vi "Dynamixel Motor Setup.vi"() -> ()   [LabVIEW 2016]
doc: "This example is designed for configuring attributes typically set on a dynamixel motor before first use."
uses:
  <instrlib>/Dynamixel Motor/Public/Motor Operation/Low Level/Alarm Setting.ctl
  <instrlib>/Dynamixel Motor/Public/Motor Operation/Low Level/Baud Setting.ctl
  <instrlib>/Dynamixel Motor/Dynamixel Motor.lvlib
panel:
  out "Searching for motor":bool
  in  "Tab Control":enum32{"Port setup", "Auto-detect settings"}(tab)
  in  "VISA resource name":refnum<visa-resource-name>
  in  "Baud rate (57600 bps)":T1=34 items=["1,000,000 bps"=1, "500,000 bps"=3, "400,000 bps"=4, "250,000 bps"=7, "200,000 bps"=9, "115200 bps"=16, "57600 bps"=34, "19200 bps"=103, "9600 bps"=207]
  in  "Force Baud Rate (True)":bool=TRUE
  in  "Search Timeout (10000 ms)":u32=10000
  in  "Starting ID (0)":u8
  in  "Ending ID (253)":u8=253
  in  "stop":bool
  out "Current angles":cluster{dbl, dbl, dbl}(knob)={0.0, 0.0, 300.0} scale=0.0..300.0
  in  "Counter-Clockwise Limit":dbl=300.0
  in  "Clockwise Limit":dbl
  out "Current Safety Limits":T2={"Temperature Limit (C)"=80, "Low Voltage Limit (V)"=6.0, "High Voltage Limit (V)"=19.0, "Maximum Torque%"=100.0} {"Maximum Torque%" min=0.0 max=100.0; "High Voltage Limit (V)" min=5.0 max=25.0; "Low Voltage Limit (V)" min=5.0 max=25.0; "Temperature Limit (C)" max=150 step=1}
  in  "Desired Safety Limits":T2={"Temperature Limit (C)"=80, "Low Voltage Limit (V)"=6.0, "High Voltage Limit (V)"=19.0, "Maximum Torque%"=100.0} {"Maximum Torque%" min=0.0 max=100.0; "High Voltage Limit (V)" min=5.0 max=25.0; "Low Voltage Limit (V)" min=5.0 max=25.0; "Temperature Limit (C)" max=150 step=1}
  in  "Apply new settings":bool
  out "Current Alarm Settings":cluster{"LED Alarm":T3, "Shutdown Alarm":T3}={"LED Alarm"={"Input Voltage"=FALSE, "Angle Limit"=FALSE, "Overheating "=TRUE, "Range"=FALSE, "Checksum"=FALSE, "Overload"=TRUE, "Instruction"=FALSE}, "Shutdown Alarm"={"Input Voltage"=FALSE, "Angle Limit"=FALSE, "Overheating "=TRUE, "Range"=FALSE, "Checksum"=FALSE, "Overload"=TRUE, "Instruction"=FALSE}}
  in  "Desired Alarm Settings":cluster{"LED Alarm":T3, "Shutdown Alarm":T3}={"LED Alarm"={"Input Voltage"=FALSE, "Angle Limit"=FALSE, "Overheating "=TRUE, "Range"=FALSE, "Checksum"=FALSE, "Overload"=TRUE, "Instruction"=FALSE}, "Shutdown Alarm"={"Input Voltage"=FALSE, "Angle Limit"=FALSE, "Overheating "=TRUE, "Range"=FALSE, "Checksum"=FALSE, "Overload"=TRUE, "Instruction"=FALSE}}
  in  "Change ID":bool
  out "Current ID":u8
  in  "New ID":u8
  # "(c) 2011-2012  National Instruments.  ALL RIGHTS RESERVED."
  # "This example is designed for \nconfiguring attributes typically set \non a Dynamixel motor before first \nuse.  \n\n1. Connect only one motor to the\nserial communications line. \n2. Choose the serial communication \nsettings and optionally the auto \ndetect settings.  \n3. Run the VI.\n4. Change the ID if desired.\n5. Enter other desired settings and\nclick Apply new settings.\n6. Stop the VI and repeat for each\nmotor you wish to configure."
  # "Clockwise Limit"
  # "Motor Position"
  # "Counter-Clockwise Limit"
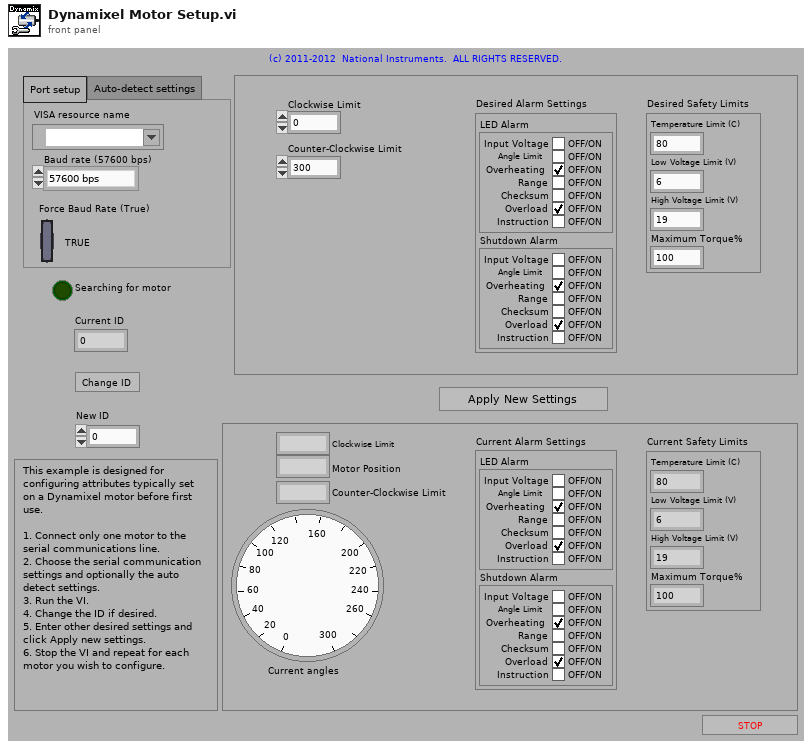
[diagram p1: front panel]
types:
  T1 = typedef "Dynamixel Motor.lvlib/Baud Setting.ctl" = u8
  T2 = cluster{"Temperature Limit (C)":u8, "Low Voltage Limit (V)":dbl, "High Voltage Limit (V)":dbl, "Maximum Torque%":dbl}
  T3 = typedef "Dynamixel Motor.lvlib/Alarm Setting.ctl" = cluster{"Input Voltage":bool, "Angle Limit":bool, "Overheating ":bool, "Range":bool, "Checksum":bool, "Overload":bool, "Instruction":bool}
  T4 = cluster{"Boolean array[0]":bool, "Boolean array[1]":bool, "Boolean array[2]":bool, "Boolean array[3]":bool, "Boolean array[4]":bool, "Boolean array[5]":bool, "Boolean array[6]":bool}
  T5 = cluster{"Boolean array":cluster{"Boolean array[0]":bool, "Boolean array[1]":bool, "Boolean array[2]":bool, "Boolean array[3]":bool, "Boolean array[4]":bool, "Boolean array[5]":bool, "Boolean array[6]":bool}, "Boolean array":cluster{"Boolean array[0]":bool, "Boolean array[1]":bool, "Boolean array[2]":bool, "Boolean array[3]":bool, "Boolean array[4]":bool, "Boolean array[5]":bool, "Boolean array[6]":bool}}
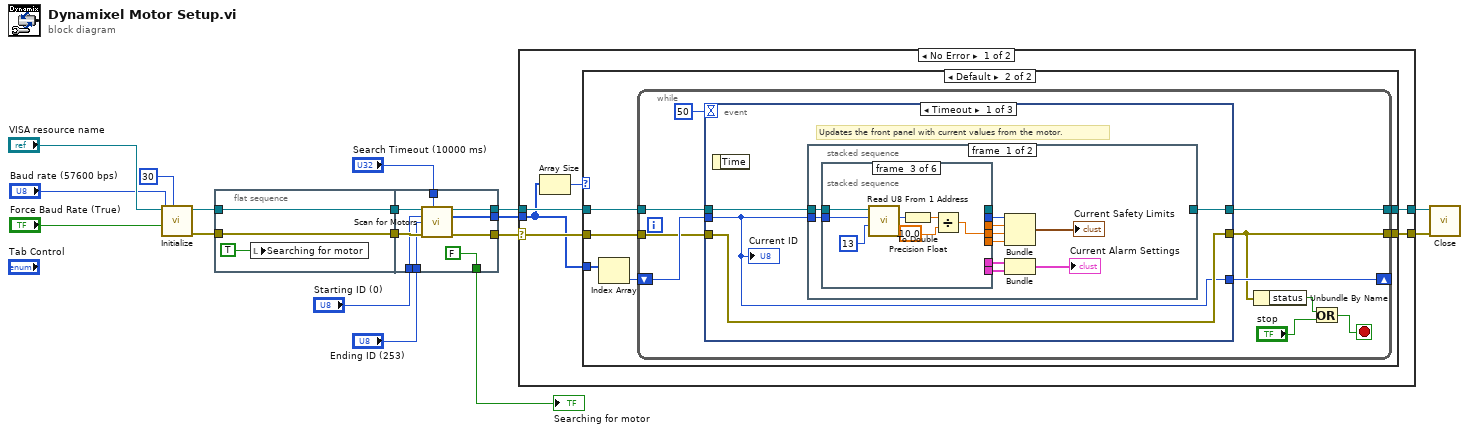
[diagram p0: block diagram]
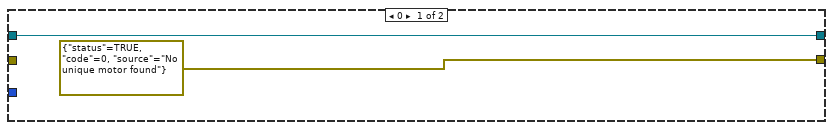
[diagram p2: hidden frame]
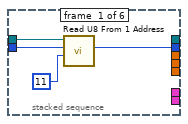
[diagram p3: hidden frame]
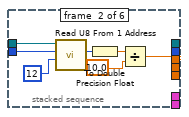
[diagram p4: hidden frame]
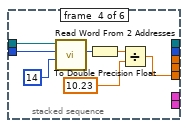
[diagram p5: hidden frame]
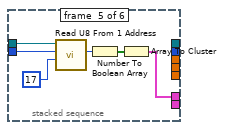
[diagram p6: hidden frame]
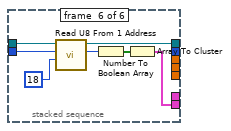
[diagram p7: hidden frame]
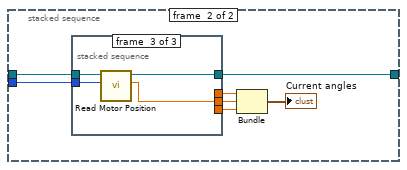
[diagram p8: hidden frame]
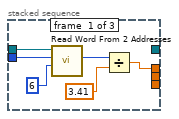
[diagram p9: hidden frame]
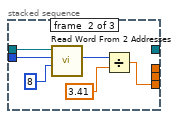
[diagram p10: hidden frame]
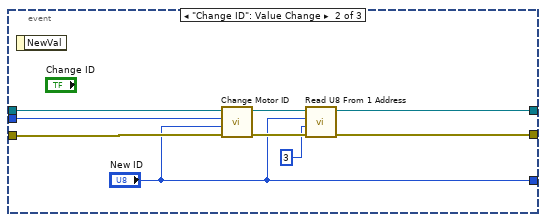
[diagram p11: hidden frame]
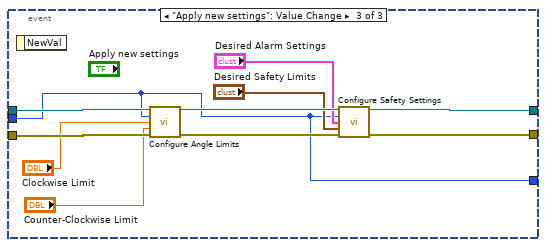
[diagram p12: hidden frame]
diagram:
  n1 = call <instrlib>:"Initialize.vi"("Timeout (30 msec)"=u32 30 ("timeout (10sec)"), "Force Baud Rate (True)"="Force Baud Rate (True)", "Baud rate (57600 bps)"="Baud rate (57600 bps)", "VISA resource name"="VISA resource name") -> ("error out"=w9:errorcluster, "VISA resource name out"=w13:refnum<visa-resource-name>)  [unwired: 6 in]
  n2 = flat-sequence {
    tunnel: w9 -> [w19]
    tunnel: w13 -> [w20]
    tunnel: [w20] -> w5
    tunnel: [w19] -> w4
    tunnel: [w28] -> w12
    tunnel: [w27] -> w11
    tunnel: [w26] -> w10
    tunnel: "Search Timeout (10000 ms)" -> [w24]
    tunnel: "Starting ID (0)" -> [w23]
    tunnel: "Ending ID (253)" -> [w22]
    tunnel: w5 -> [w29]
    tunnel: w4 -> [w25]
    tunnel: [FALSE ("Searching for motor")] -> w3
    frame #0 {
      n3 = local write "Searching for motor"(TRUE ("Searching for motor")) -> ()
    }
    frame #1 {
      n4 = call <instrlib>:"Scan for Motors.vi"("VISA resource name"=w29, "Starting ID (0)"=w23, "Ending ID (253)"=w22, "Search Timeout (10000 ms)"=w24, "error in (no error)"=w25) -> ("VISA resource name out"=w28:refnum<visa-resource-name>, "Motors IDs Found"=w26:u8[], "error out"=w27:errorcluster)  [unwired: 8 in]
    }
  }
  n5 = case shown="No Error" w11 {
    selector: w11 -> [w33 w149]
    tunnel: [w35 w150] -> w17
    tunnel: w12 -> [w34 w150]
    tunnel: [w32 w149] -> w14
    tunnel: w10 -> [w31 _]
    frame No Error {
      n6 = Array Size(array=w31) -> (size(s)=w30:i32)
      n7 = case shown="Default" w30 {
        tunnel: [w37 w43] -> w35
        tunnel: w34 -> [w37 w42]
        tunnel: w33 -> [_ w41]
        tunnel: w31 -> [_ w40]
        tunnel: [errorcluster {"status"=TRUE, "code"=0, "source"="No unique motor found"} ("error out") w38] -> w32
        frame 0 {
        }
        frame Default {
          n8 = Index Array(array=w40) -> (element=w39:u8)  [unwired: 1 in]
          n9 = while {
            tunnel: w41 -> [w49]
            shift-right: [w48] -> _
            shift-left: w39 -> [w51]
            tunnel: w42 -> [w52]
            tunnel: [w50] -> w43
            tunnel: [w47] -> w38
            stop <- w46 stop-if-true
            n10 = event shown="[0] Timeout" {
              selector: _ -> [_ _ _]
              dyn-events: _ -> [_ _ _]
              timeout: 50 -> [_ _ _]
              tunnel: w52 -> [w57 w137 w148]
              tunnel: w51 -> [w54 w132 w138]
              tunnel: [w56 w135 w145] -> w50
              tunnel: w49 -> [w55 w133 w147]
              tunnel: [w55 w131 w143] -> w47
              tunnel: [w54 "New ID" w138] -> w48
              event Timeout {
                # "Updates the front panel with current values from the motor."
                n11 = event-data() -> ()  [unwired: 1 in, 1 out]
                n12 = stacked-sequence {
                  tunnel: w57 -> [w65 w108]
                  tunnel: w54 -> [w58 w107]
                  tunnel: [_ w106] -> w56
                  frame #0 {
                    n13 = stacked-sequence {
                      tunnel: w65 -> [w71 w78 w85 w92 w98 w105]
                      tunnel: [w70 _ _ _ _ _] -> w64
                      tunnel: [_ w74 _ _ _ _] -> w63
                      tunnel: [_ _ w81 _ _ _] -> w62
                      tunnel: [_ _ _ w88 _ _] -> w61
                      tunnel: [_ _ _ _ w95 _] -> w60
                      tunnel: [_ _ _ _ _ w102] -> w59
                      tunnel: [_ _ _ _ _ w101] -> _
                      tunnel: w58 -> [w68 w72 w79 w86 w93 w99]
                      frame #0 {
                        n14 = call <instrlib>:"Read U8 From 1 Address.vi"("Address number (0)"=u8 11 ("Address # DEC"), "Motor ID (0)"=w68, "VISA resource name"=w71) -> ("Data"=w70:u8)  [unwired: 6 in, 2 out]
                      }
                      frame #1 {
                        n15 = call <instrlib>:"Read U8 From 1 Address.vi"("Address number (0)"=u8 12 ("Address # DEC"), "Motor ID (0)"=w72, "VISA resource name"=w78) -> ("Data"=w77:u8)  [unwired: 6 in, 2 out]
                        n16 = To Double Precision Float(number=w77) -> (double precision float=w76:dbl)
                        n17 = Divide(x=w76, y=10.0) -> (x/y=w74:dbl)
                      }
                      frame #2 {
                        n18 = call <instrlib>:"Read U8 From 1 Address.vi"("Address number (0)"=u8 13 ("Address # DEC"), "Motor ID (0)"=w79, "VISA resource name"=w85) -> ("Data"=w84:u8)  [unwired: 6 in, 2 out]
                        n19 = To Double Precision Float(number=w84) -> (double precision float=w83:dbl)
                        n20 = Divide(x=w83, y=10.0) -> (x/y=w81:dbl)
                      }
                      frame #3 {
                        n21 = call <instrlib>:"Read Word From 2 Addresses.vi"("Address number (0)"=u8 14 ("Address # DEC"), "Motor ID (0)"=w86, "VISA resource name"=w92) -> ("Data"=w91:u16)  [unwired: 6 in, 2 out]
                        n22 = To Double Precision Float(number=w91) -> (double precision float=w90:dbl)
                        n23 = Divide(x=w90, y=10.23) -> (x/y=w88:dbl)
                      }
                      frame #4 {
                        n24 = call <instrlib>:"Read U8 From 1 Address.vi"("Address number (0)"=u8 17 ("Address # DEC"), "Motor ID (0)"=w93, "VISA resource name"=w98) -> ("Data"=w96:u8)  [unwired: 6 in, 2 out]
                        n25 = Number To Boolean Array(number=w96) -> (Boolean array=w97:bool[])
                        n26 = Array To Cluster(array=w97) -> (cluster=w95:T4)
                      }
                      frame #5 {
                        n27 = call <instrlib>:"Read U8 From 1 Address.vi"("Address number (0)"=u8 18 ("Address # DEC"), "Motor ID (0)"=w99, "VISA resource name"=w105) -> ("Data"=w103:u8, "VISA resource name out"=w101:refnum<visa-resource-name>)  [unwired: 6 in, 1 out]
                        n28 = Number To Boolean Array(number=w103) -> (Boolean array=w104:bool[])
                        n29 = Array To Cluster(array=w104) -> (cluster=w102:T4)
                      }
                    }
                    n30 = Bundle("Data"=w64, w63, w62, w61) -> (→"Current Safety Limits":cluster{"Data":u8, dbl, dbl, dbl})  [unwired: 1 in]
                    n31 = Bundle("Boolean array"=w60, "Boolean array"=w59) -> (→"Current Alarm Settings":T5)  [unwired: 1 in]
                  }
                  frame #1 {
                    n32 = stacked-sequence {
                      tunnel: w108 -> [w118 w124 w128]
                      tunnel: w107 -> [w114 w120 w127]
                      tunnel: [w115 _ _] -> w111
                      tunnel: [_ _ w126] -> w110
                      tunnel: [_ w121 _] -> w109
                      tunnel: [_ _ w125] -> w106
                      frame #0 {
                        n33 = call <instrlib>:"Read Word From 2 Addresses.vi"("Address number (0)"=u8 6 ("Address # DEC"), "Motor ID (0)"=w114, "VISA resource name"=w118) -> ("Data"=w116:u16)  [unwired: 6 in, 2 out]
                        n34 = Divide(x=w116, y=3.41) -> (x/y=w115:dbl)
                      }
                      frame #1 {
                        n35 = call <instrlib>:"Read Word From 2 Addresses.vi"("Address number (0)"=u8 8 ("Address # DEC"), "Motor ID (0)"=w120, "VISA resource name"=w124) -> ("Data"=w122:u16)  [unwired: 6 in, 2 out]
                        n36 = Divide(x=w122, y=3.41) -> (x/y=w121:dbl)
                      }
                      frame #2 {
                        n37 = call <instrlib>:"Read Motor Position.vi"("Motor ID (0)"=w127, "VISA resource name"=w128) -> ("Position (deg)"=w126:dbl, "VISA resource name out"=w125:refnum<visa-resource-name>)  [unwired: 7 in, 1 out]
                      }
                    }
                    n38 = Bundle(w111, "Position (deg)"=w110, w109) -> (→"Current angles":cluster{dbl, "Position (deg)":dbl, dbl})  [unwired: 1 in]
                  }
                }
                "Current ID" <- w54
              }
              event "Change ID": Value Change {
                n39 = event-data() -> ()  [unwired: 1 in, 1 out]
                n40 = call <instrlib>:"Change Motor ID.vi"("error in (no error)"=w133, "New ID"="New ID", "Current ID"=w132, "VISA resource name"=w137) -> ("error out"=w134:errorcluster, "VISA Resource Out"=w136:refnum<visa-resource-name>)  [unwired: 6 in]
                n41 = call <instrlib>:"Read U8 From 1 Address.vi"("Error in (no error)"=w134, "Address number (0)"=u8 3 ("Address number (dec)"), "Motor ID (0)"="New ID", "VISA resource name"=w136) -> ("error out"=w131:errorcluster, "VISA resource name out"=w135:refnum<visa-resource-name>)  [unwired: 5 in, 1 out]
              }
              event "Apply new settings": Value Change {
                n42 = event-data() -> ()  [unwired: 1 in, 1 out]
                n43 = call <instrlib>:"Configure Angle Limits.vi"("VISA resource name"=w148, "Motor ID (0)"=w138, "Clockwise Angle Limit (0 deg)"="Clockwise Limit", "Counter-Clockwise Angle Limit (300 deg)"="Counter-Clockwise Limit", "error in (no error)"=w147) -> ("VISA resource name out"=w146:refnum<visa-resource-name>, "error out"=w144:errorcluster)  [unwired: 9 in]
                n44 = call <instrlib>:"Configure Safety Settings.vi"("VISA resource name"=w146, "Motor ID (0)"=w138, "Alarm Settings"="Desired Alarm Settings", "Safety Limits"="Desired Safety Limits", "error in (no error)"=w144) -> ("VISA resource name out"=w145:refnum<visa-resource-name>, "error out"=w143:errorcluster)  [unwired: 9 in]
              }
            }
            n45 = Unbundle By Name(w47) -> ("status"=w45:bool)
            n46 = Or(x=w45, y="stop") -> (x .or. y?=w46:bool)
          }
        }
      }
    }
    frame Error {
    }
  }
  n47 = call <instrlib>:"Close.vi"("error in (no error)"=w14, "VISA resource name"=w17) -> ()  [unwired: 9 in, 1 out]
  "Searching for motor" <- w3
